vi "LED Lights Subsystem.vi"(8 "error in":errorcluster) -> ()   [LabVIEW 2015]
uses:
  <vilib>/Rock Robotics/SystemInterfaces/i2clib/i2c_bus.ctl
panel:
  in  "Send":bool
  in  "Light ID":u8=3
  in  "Blue":u8=153
  in  "Green":u8=12
  in  "Red":u8=64
  out "error out":errorcluster
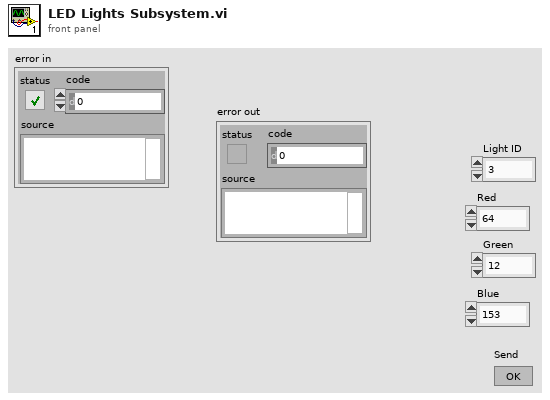
[diagram p1: front panel]
types:
  T1 = typedef "i2c_bus.ctl" = enum16{"I2C On-Board", "I2C MXP", "Invalid"}
  T2 = typedef "LED Lights Ref.ctl" = cluster{"I2CDevRef":T3}
  T3 = typedef "WPI_I2CDevRef.ctl" = cluster{"DevStatus":errorcluster, "Device Address":u8, "Handle":i32, "I2C Bus":T1}
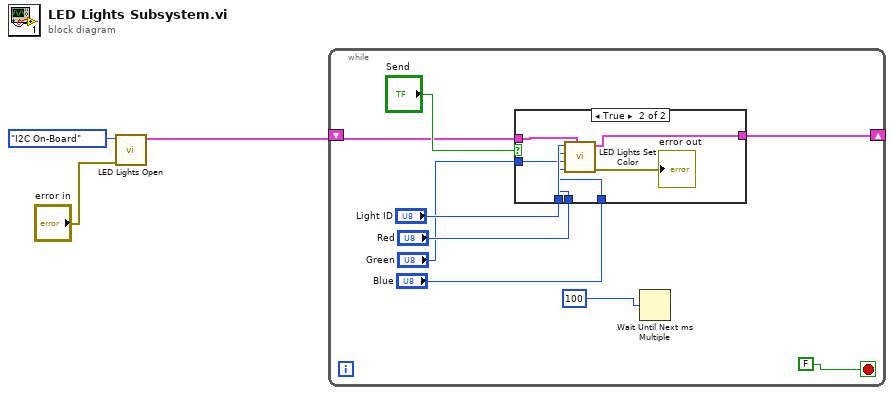
[diagram p0: block diagram]
diagram:
  n1 = call "LED Lights Open.vi"("error in"="error in", "I2C Bus"=i2c_bus."I2C On-Board") -> ("output cluster"=w2:T2)  [unwired: 8 in, 1 out]
  n2 = while {
    shift-right: [w4] -> _
    shift-left: w2 -> [w9]
    stop <- FALSE stop-if-true
    n3 = case shown="True" "Send" {
      tunnel: w9 -> [w13 w20]
      tunnel: "Light ID" -> [_ w19]
      tunnel: "Red" -> [_ w18]
      tunnel: "Green" -> [_ w17]
      tunnel: "Blue" -> [_ w16]
      tunnel: [w13 w14] -> w4
      frame False {
      }
      frame True {
        n4 = call "LED Lights Set Color.vi"("LED Lights Ref In"=w20, "Blue"=w16, "Green"=w17, "Red"=w18, "Light ID"=w19) -> ("error out"=→"error out":errorcluster, "LED Lights Ref Out"=w14:T2)  [unwired: 5 in]
      }
    }
    n5 = Wait Until Next ms Multiple(millisecond multiple=100) -> ()  [unwired: 1 out]
  }
